vi "Dialog Macro Error Description.vi"(8 "Error In":errorcluster, 9 "Warning?":bool, 10 "Error?":bool, 11 "Error Description IN":string) -> (0 "Error Out":errorcluster)   [LabVIEW 2012]
doc: "SciScan 1.2 160622"
panel:
  out "Error Description Displayed":string caption="Error Description"
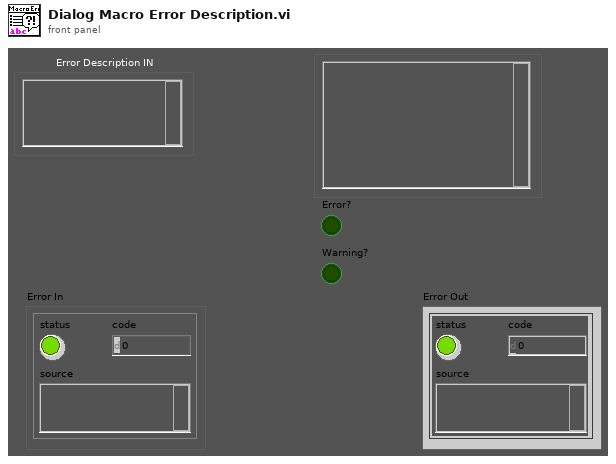
[diagram p1: front panel]
types:
  T1 = enum32{"Invalid", "Default", "Floating", "Floating/Auto-Hide", "Modal"}
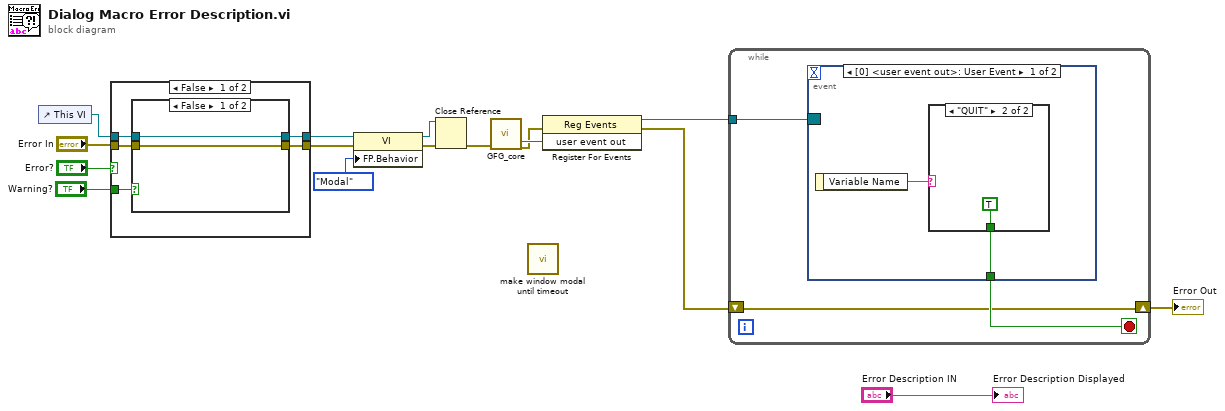
[diagram p0: block diagram]
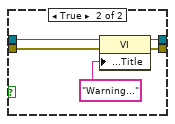
[diagram p2: hidden frame]
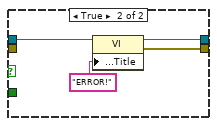
[diagram p3: hidden frame]
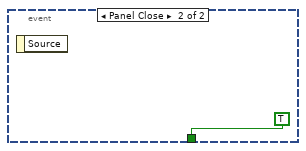
[diagram p5: hidden frame]
diagram:
  n1 = control-ref of="This VI"() -> (w5:refnum<vi>)
  n2 = case shown="False" "Error?" {
    tunnel: w5 -> [w20 w32]
    tunnel: "Warning?" -> [w21 _]
    tunnel: [w19 w30] -> w2
    tunnel: "Error In" -> [w18 _]
    tunnel: [w17 w29] -> w1
    frame False {
      n3 = case shown="False" w21 {
        tunnel: w20 -> [w22 w27]
        tunnel: [w23 w26] -> w19
        tunnel: w18 -> [w23 w25]
        tunnel: [w22 w24] -> w17
        frame False {
        }
        frame True {
          n4 = property class="VI"(reference=w27, error in=w25, "Front Panel.Title"="Warning..." ("Front Panel Window:Title")) -> (reference out=w24:refnum<vi>, error out=w26:errorcluster)
        }
      }
    }
    frame True {
      n5 = property class="VI"(reference=w32, "Front Panel.Title"="ERROR!" ("Front Panel Window:Title")) -> (reference out=w29:refnum<vi>, error out=w30:errorcluster)  [unwired: 1 in]
    }
  }
  n6 = property class="VI"(reference=w1, error in=w2, "FP.Behavior"=T1."Modal" ("Front Panel Window:Behavior")) -> (reference out=w11:refnum<vi>, error out=w12:errorcluster)
  n7 = Close Reference(reference=w11, error in (no error)=w12) -> (error out=w10:errorcluster)
  n8 = call "GFG_core.vi"("error in (no error)"=w10) -> ("user event out"=w16:refnum<user-event>, "error out"=w15:errorcluster)  [unwired: 12 in, 5 out]
  n9 = call "make window modal until timeout.vi"() -> ()  [unwired: 12 in]
  n10 = register-events(error in=w15, w16) -> (reference out=w14:refnum<event-registration>, error out=w8:errorcluster)  [unwired: 1 in]
  n11 = while {
    tunnel: w14 -> [w35]
    shift-right: [w33] -> w7
    shift-left: w8 -> [w33]
    stop <- w34 stop-if-true
    n12 = event shown="[0] <user event out>: User Event" {
      selector: w35 -> [_ _]
      dyn-events: _ -> [_ _]
      timeout: _ -> [_ _]
      tunnel: [w36 TRUE] -> w34
      event User Event {
        n13 = event-data() -> ("Variable Name"=w37:string)  [unwired: 1 in]
        n14 = case shown="\"QUIT\"" w37 {
          tunnel: [_ TRUE] -> w36
          frame Default {
          }
          frame "QUIT" {
          }
        }
      }
      event Panel Close {
        n15 = event-data() -> ()  [unwired: 1 in, 1 out]
      }
    }
  }
  "Error Out" <- w7
  "Error Description Displayed" <- "Error Description IN"
